vi "Block Float (U32).vi"(8 "Input Valid":bool=TRUE, 10 "Binary Number 2":u32 format="%.0b", 11 "Binary Number 1":u32 format="%032b") -> (0 "Output Valid":bool=TRUE, 2 "Block Float Mantissa 2":u32 format="%032b", 3 "Block Float Mantissa 1":u32 format="%032b", 5 "Common Exponent":i8)   [LabVIEW 2010]
doc: "This VI computes the block floating point representation of two numbers"
panel:
  # "Check:\na) If Input1=0\nb)If Input2=0\nc)If Input1 and2=0\nc)If Input1 and 2!=0"
  # "This code is a untested code"
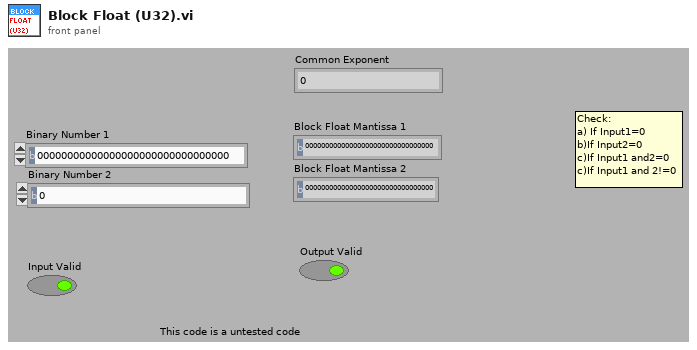
[diagram p1: front panel]
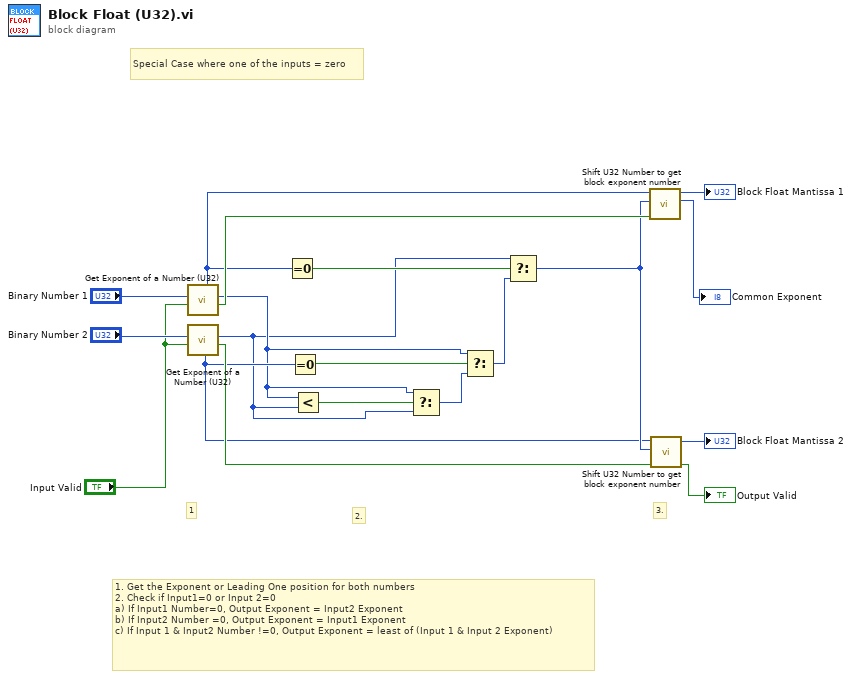
[diagram p0: block diagram]
diagram:
  # "1. Get the Exponent or Leading One position for both numbers\n2. Check if Input1=0 or Input 2=0\na) If Input1 Number=0, Output Exponent = Input2 Exponent\nb) If Input2 Number =0, Output Exponent = Input1 Exponent\nc) If Input 1 & Input2 Number !=0, Output Exponent = least of (Input 1 & Input 2 Exponent)"
  # "3."
  # "2."
  # "1"
  # "Special Case where one of the inputs = zero"
  n1 = call "Get Exponent of a Number (U32).vi"("Input Valid"="Input Valid", "Binary Number"="Binary Number 1") -> ("Output Valid"=w16:bool, "Exponent"=w2:u8, "Binary Number"=w4:u32)  [unwired: 7 in]
  n2 = call "Get Exponent of a Number (U32).vi"("Input Valid"="Input Valid", "Binary Number"="Binary Number 2") -> ("Output Valid"=w19:bool, "Exponent"=w1:u8, "Binary Number"=w3:u32)  [unwired: 7 in]
  n3 = Equal To 0?(x=w4) -> (x = 0?=w10:bool)
  n4 = Equal To 0?(x=w3) -> (x = 0?=w9:bool)
  n5 = Less?(x=w2, y=w1) -> (x < y?=w11:bool)
  n6 = Select(t=w2, s=w11, f=w1) -> (s? t:f=w8:u8)
  n7 = Select(t=w2, s=w9, f=w8) -> (s? t:f=w7:u8)
  n8 = Select(t=w1, s=w10, f=w7) -> (s? t:f=w6:u8)
  n9 = call "Shift U32 Number to get block exponent number.vi"("Input Valid"=w16, "Leading Zero Position"=w6, "Binary Number"=w4) -> ("Block Float Exponent"=→"Common Exponent":i8, "Block Float Mantissa"=→"Block Float Mantissa 1":u32)  [unwired: 6 in, 1 out]
  n10 = call "Shift U32 Number to get block exponent number.vi"("Input Valid"=w19, "Leading Zero Position"=w6, "Binary Number"=w3) -> ("Output Valid"=→"Output Valid":bool, "Block Float Mantissa"=→"Block Float Mantissa 2":u32)  [unwired: 6 in, 1 out]
